vi "ADIS16448 Loop.vi"(8 "error in":errorcluster) -> ()   [LabVIEW 2019]
uses:
  Typedef/ADIS16448 Device Reference.ctl
  Typedef/ADIS16448 Hardware Configuration.ctl
  <vilib>/Rock Robotics/WPI/SPI/WPI_SPIMode.ctl
  <vilib>/Rock Robotics/SystemInterfaces/DIO/FPGA_DIOChannel.ctl
  <vilib>/Rock Robotics/SystemInterfaces/spilib/spi_bus.ctl
  Typedef/ADIS16448 Status.ctl
  Typedef/ADIS16448 Data.ctl
  Typedef/ADIS16448 Process.ctl
  Typedef/ADIS16448 Command Type.ctl
  <vilib>/Rock Robotics/SystemInterfaces/CounterEncoderSourceConvertion/FPGA_CounterEncoderSourceConvertionLVSourceType.ctl
  <vilib>/Rock Robotics/SystemInterfaces/DIO/FPGA_DIODigitalSourceChannel.ctl
  <vilib>/Rock Robotics/SystemInterfaces/AnalogTrigger/FPGA_AnalogTriggerIndex.ctl
  <vilib>/Rock Robotics/SystemInterfaces/AnalogTrigger/FPGA_AnalogTriggerOutType.ctl
  Typedef/ADIS16448 Calibration Time.ctl
  <vilib>/Rock Robotics/WPI/SPI/WPI_SPIDevRef.ctl
  Typedef/ADIS16448 Register.ctl
  <vilib>/Rock Robotics/WPI/Counter/WPI_CounterDigitalInputToDigitalSource.vi
  <vilib>/Rock Robotics/SystemInterfaces/Utilities/FPGA_UtilitiesRead LocalTime.vi
  <vilib>/ptbypt/NI_PtbyPt.lvlib
panel:
  in  "Calibration Time":T1
  in  "element":T2
  out "Waveform Chart":dbl(graph)
  in  "ADIS16448DevRef":T3={"DevStatus"={"status"=FALSE, "code"=0, "source"=""}, "Hardware Config"={"SPI Clock Rate (Hz)"=1000000.0, "IMU SPI Mode (3)"=enum."Mode 3 (Clk Idle High,Sample on Trailing)", "IMU Reset Pin"=enum."SPI Port CS2", "IMU SPI Bus"=enum."SPI On-Board, CS0", "IMU Data Ready Pin"=enum."SPI Port CS1", "Stall Config"={"Pow2BytesPerRead"=255, "StallTicks"=640, "CsToSclkTicks"=5}, "IMU Status LED Pin"=enum."DIO MXP 9"}, "Calibration Complete"=refnum, "Status FIFO"=refnum, "Last Value Reference"=refnum, "Sychronous Process VI"=refnum, "Cmd FIFO"=refnum, "Source"={"DevStatus"={"status"=FALSE, "code"=0, "source"=""}, "AnalogTriggerMode?"=FALSE, "DigitalMode"={"DIO Channel"=enum."Disabled"}, "AnalogTriggerMode"={"AnalogTriggerIndex"=enum."Trig 0", "OutputType"=enum."InWindow"}}, "Data FIFO"=refnum, "IMU Status LED Pin"=enum."DIO MXP 9", "Calibration Time"=5}
  in  "Main Name":string
  # "XG_BIAS_LOW"
  # "XG_BIAS_HIGH"
  # "YG_BIAS_LOW"
  # "YG_BIAS_HIGH"
  # "ZG_BIAS_LOW"
  # "ZG_BIAS_HIGH"
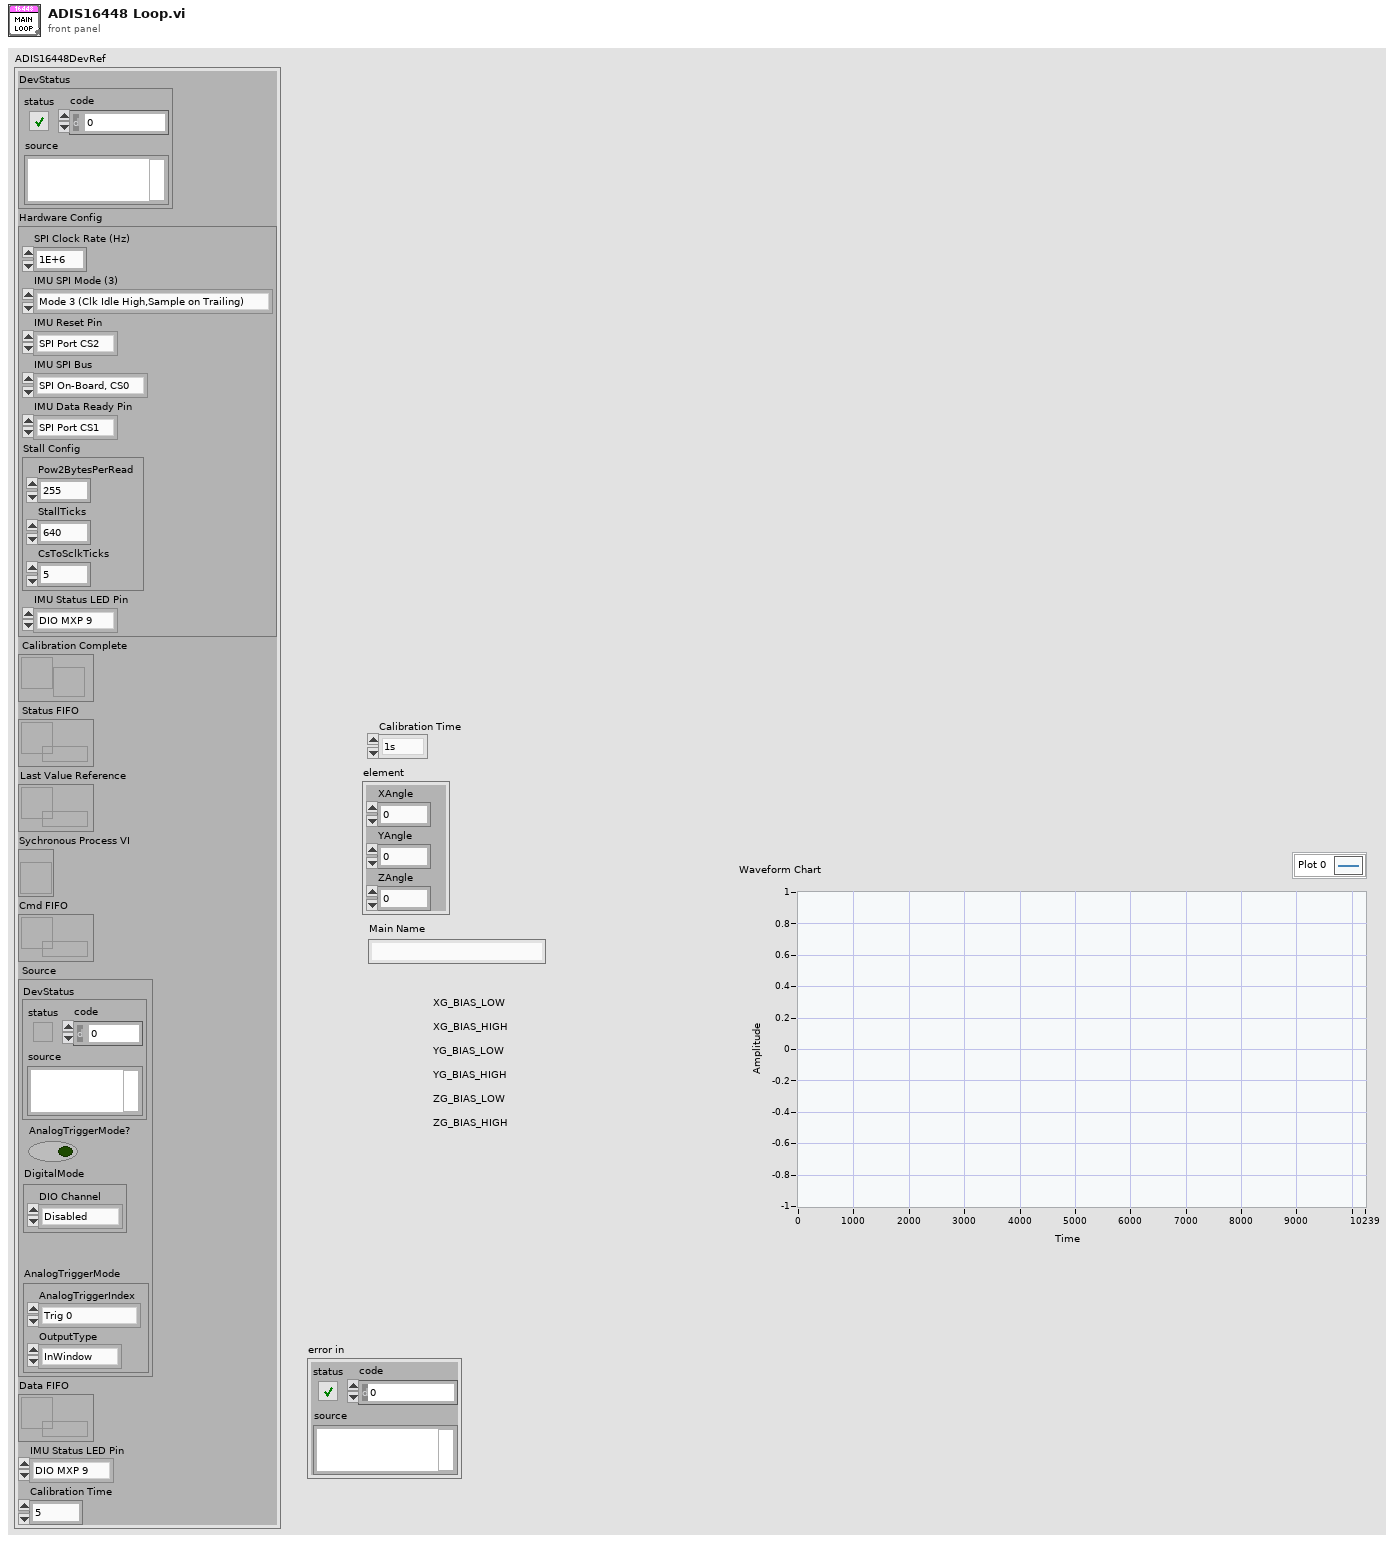
[diagram p1: front panel]
types:
  T1 = typedef "ADIS16448 Calibration Time.ctl" = enum16{"1s", "s", "4.9ms", "9.8ms", "19.5ms", "39.1ms", "78.1ms", "156.3ms", "312.5ms", "625ms", "1.25s", "2.5s", "5s", "10s", "20s", "40s", "80s", "160s", "320s"}
  T2 = typedef "ADIS16448 Data.ctl" = cluster{"XAngle":dbl, "YAngle":dbl, "ZAngle":dbl}
  T3 = typedef "ADIS16448 Device Reference.ctl" = cluster{"DevStatus":errorcluster, "Hardware Config":T4, "Calibration Complete":refnum<notifier>, "Status FIFO":refnum<k33>, "Last Value Reference":refnum<data-value>, "Sychronous Process VI":T8, "Cmd FIFO":refnum<k33>, "Source":T9, "Data FIFO":refnum<k33>, "IMU Status LED Pin":T6, "Calibration Time":i32}
  T4 = typedef "ADIS16448 Hardware Configuration.ctl" = cluster{"SPI Clock Rate (Hz)":dbl, "IMU SPI Mode (3)":T5, "IMU Reset Pin":T6, "IMU SPI Bus":T7, "IMU Data Ready Pin":T6, "Stall Config":cluster{"Pow2BytesPerRead":u8, "StallTicks":u16, "CsToSclkTicks":u8}, "IMU Status LED Pin":T6}
  T5 = typedef "WPI_SPIMode.ctl" = enum16{"Mode 0 (Clk Idle Low,Sample on Leading)", "Mode 1 (Clk Idle Low,Sample on Trailing)", "Mode 2 (Clk Idle High,Sample on Leading)", "Mode 3 (Clk Idle High,Sample on Trailing)"}
  T6 = typedef "FPGA_DIOChannel.ctl" = enum8{"DIO 0", "DIO 1", "DIO 2", "DIO 3", "DIO 4", "DIO 5", "DIO 6", "DIO 7", "DIO 8", "DIO 9", "DIO MXP 0", "DIO MXP 1", "DIO MXP 2", "DIO MXP 3", "DIO MXP 4", "DIO MXP 5", "DIO MXP 6", "DIO MXP 7", "DIO MXP 8", "DIO MXP 9", "DIO MXP 10", "DIO MXP 11", "DIO MXP 12", "DIO MXP 13", "DIO MXP 14", "DIO MXP 15", "SPI Port CS1", "SPI Port CS2", "SPI Port CS3", "SPI Port MISO", "SPI Port MOSI", "Invalid"}
  T7 = typedef "spi_bus.ctl" = enum16{"SPI On-Board, CS0", "SPI On-Board, CS1", "SPI On-Board, CS2", "SPI On-Board, CS3", "SPI MXP", "Invalid"}
  T8 = typedef "ADIS16448 Process.ctl" = refnum<vi>
  T9 = typedef "FPGA_CounterEncoderSourceConvertionLVSourceType.ctl" = cluster{"DevStatus":errorcluster, "AnalogTriggerMode?":bool, "DigitalMode":cluster{"DIO Channel":T10}, "AnalogTriggerMode":cluster{"AnalogTriggerIndex":T11, "OutputType":T12}}
  T10 = typedef "FPGA_DIODigitalSourceChannel.ctl" = enum8{"DIO 0", "DIO 1", "DIO 2", "DIO 3", "DIO 4", "DIO 5", "DIO 6", "DIO 7", "DIO 8", "DIO 9", "DIO MXP 0", "DIO MXP 1", "DIO MXP 2", "DIO MXP 3", "DIO MXP 4", "DIO MXP 5", "DIO MXP 6", "DIO MXP 7", "DIO MXP 8", "DIO MXP 9", "DIO MXP 10", "DIO MXP 11", "DIO MXP 12", "DIO MXP 13", "DIO MXP 14", "DIO MXP 15", "SPI Port CS1", "SPI Port CS2", "SPI Port CS3", "SPI Port MISO", "SPI Port MOSI", "Disabled"}
  T11 = typedef "FPGA_AnalogTriggerIndex.ctl" = enum8{"Trig 0", "Trig 1", "Trig 2", "Trig 3", "Trig 4", "Trig 5", "Trig 6", "Trig 7", "Invalid"}
  T12 = typedef "FPGA_AnalogTriggerOutType.ctl" = enum16{"InWindow", "TriggerState", "Rising", "Falling"}
  T13 = typedef "WPI_SPIDevRef.ctl" = cluster{"DevStatus":errorcluster, "Handle":i32, "SPI Bus":T7}
  T14 = cluster{"SPIDevRef":T13, "Data Counter":u16, "Reset":bool, "Digital Source":T9, "Bytes Per Sample":u32, "Data":dbl[], "ADIS16448DevRef":T3, "TimeStampPrev":u32, "Sensor to Robot Rotation":dbl[][], "AutoSPI Active?":bool, "Offsets":dbl[], "Offset Counter":i32, "Data Header":u8[], "Zero Byte Count":u8, "AutoSPI Override":bool}
  T15 = typedef "ADIS16448 Status.ctl" = cluster{"Calibrated?":bool}
  T16 = typedef "ADIS16448 Register.ctl" = u8
  T17 = typedef "ADIS16448 Command Type.ctl" = cluster{"Command":enum16{"None", "Reset", "Rewrite Config", "Start Recal", "Recalibrate", "Recal Complete", "Exit Auto SPI", "Start Auto SPI"}, "Data":u32}
  T18 = typedef "WPI_DigitalOutputDevRef.ctl" = cluster{"DIO Channel":T6, "DevStatus":errorcluster}
  T19 = typedef "WPI_DigitalInputDevRef.ctl" = cluster{"DevStatus":errorcluster, "DIO Channel":T6}
  T20 = cluster{"Pow2BytesPerRead":u8, "StallTicks":u16, "CsToSclkTicks":u8}
  T21 = enum16{"None", "Reset", "Rewrite Config", "Start Recal", "Recalibrate", "Recal Complete", "Exit Auto SPI", "Start Auto SPI"}
  T22 = enum32{"Bad", "Idle", "Run top level", "Running"}
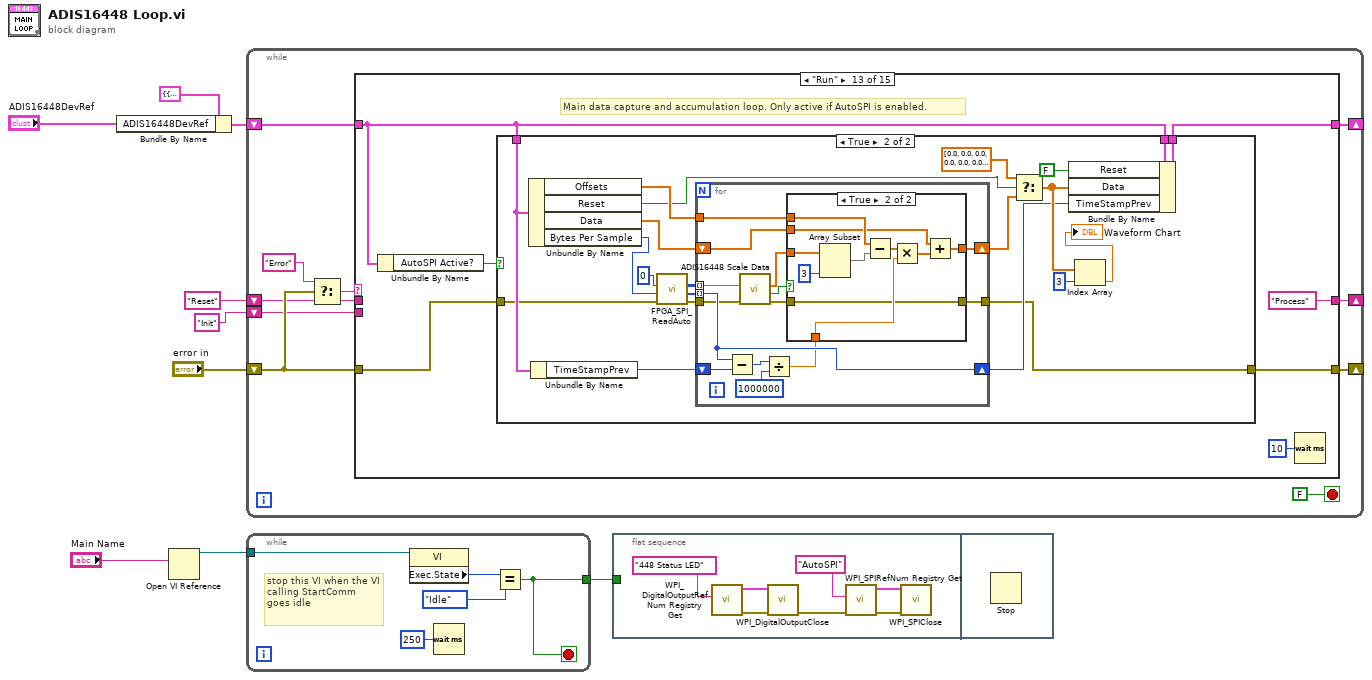
[diagram p0: block diagram]
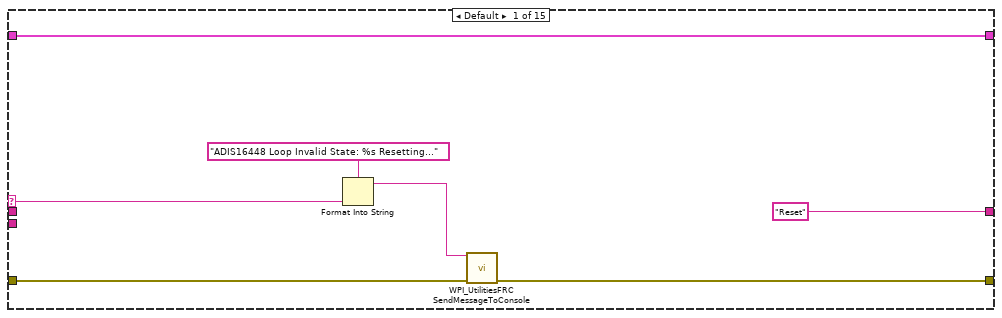
[diagram p2: hidden frame]
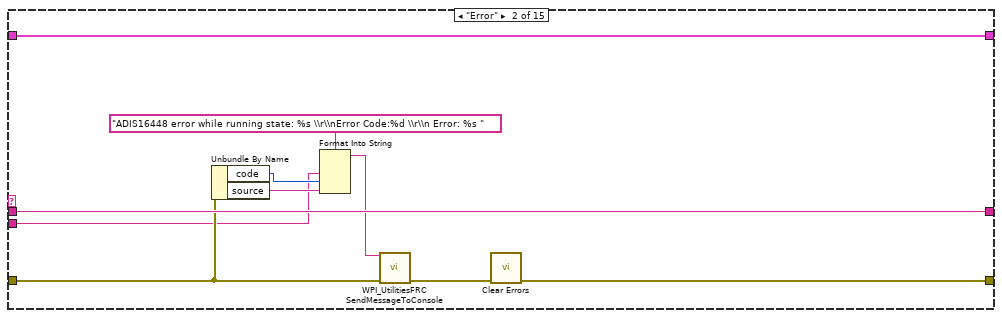
[diagram p3: hidden frame]
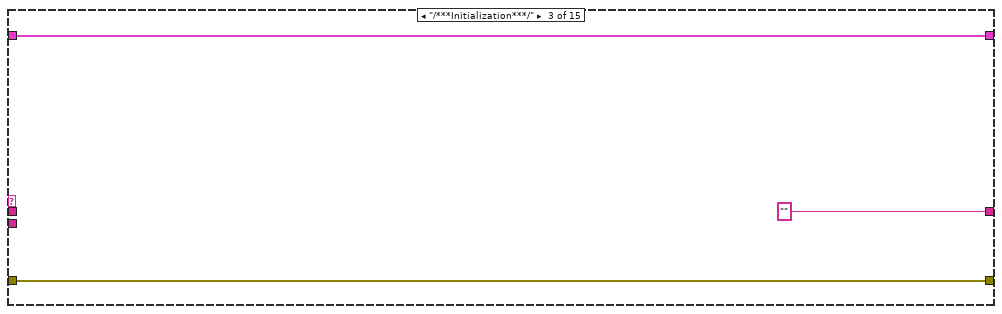
[diagram p4: hidden frame]
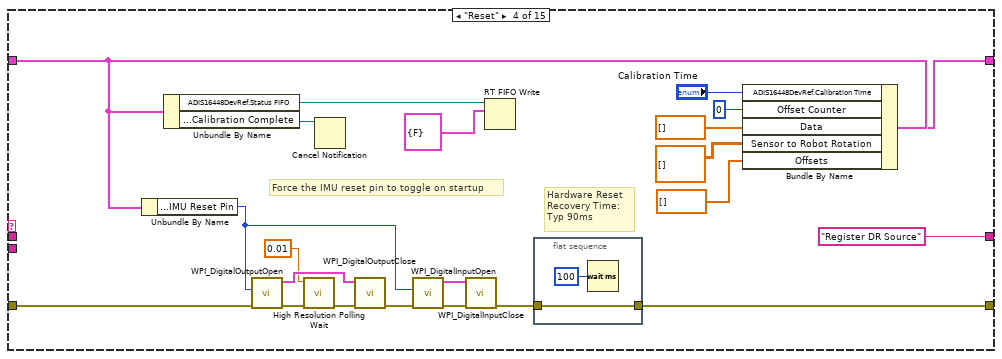
[diagram p5: hidden frame]
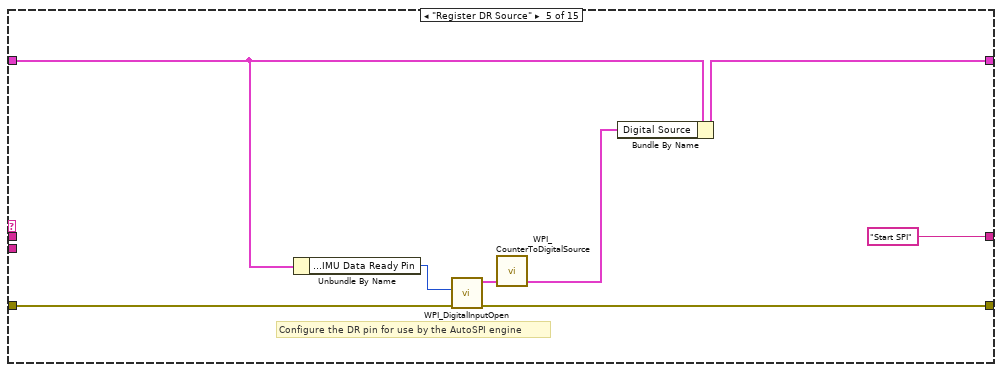
[diagram p6: hidden frame]
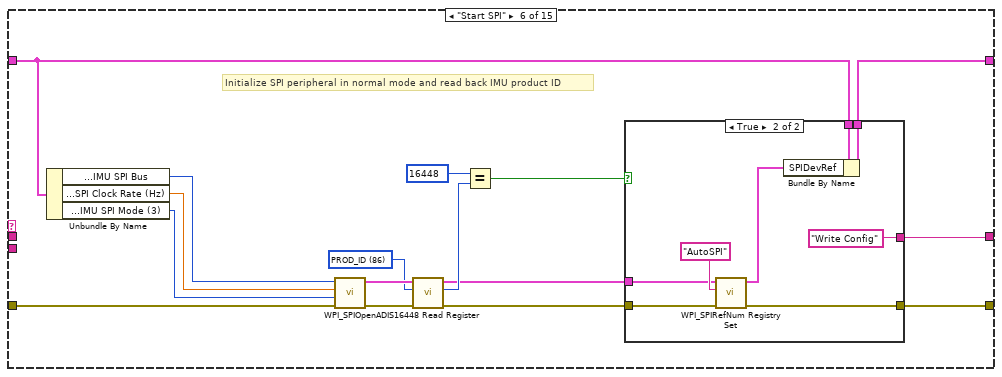
[diagram p7: hidden frame]
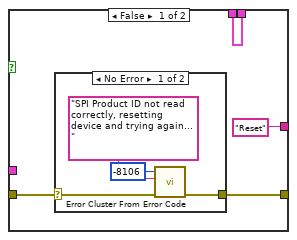
[diagram p8: hidden frame]
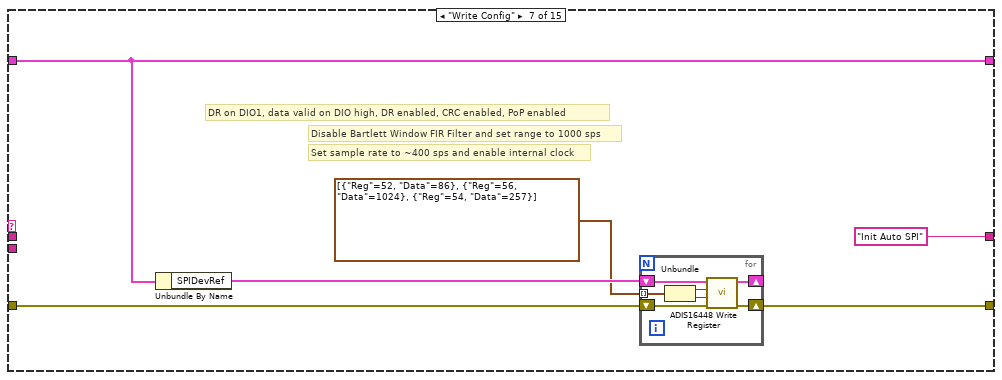
[diagram p10: hidden frame]
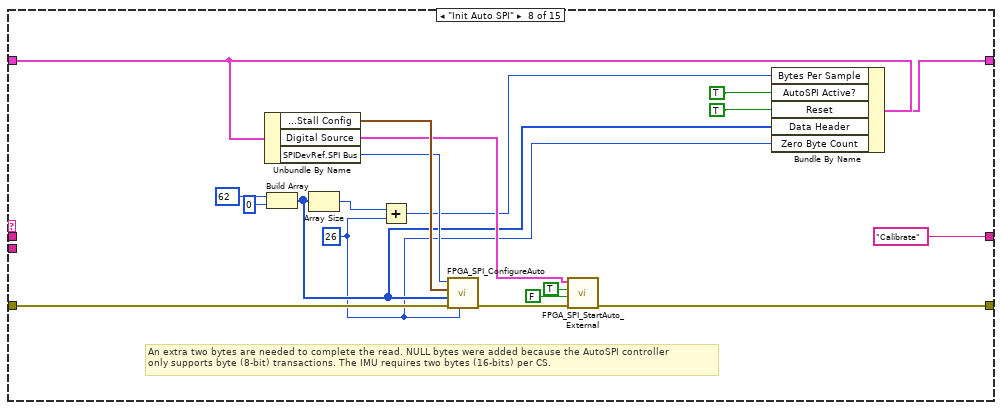
[diagram p11: hidden frame]
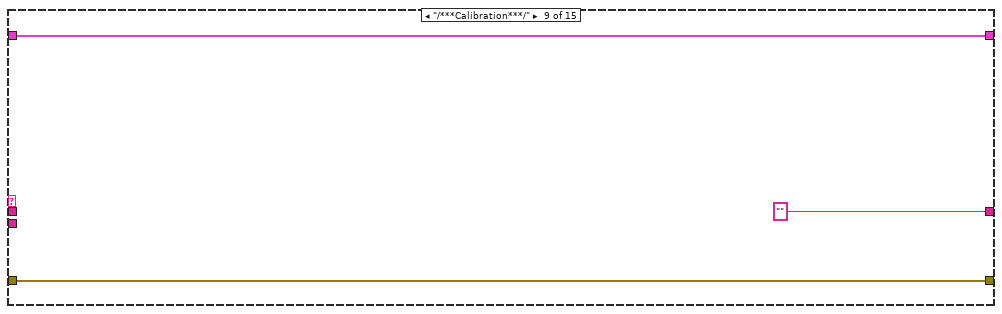
[diagram p12: hidden frame]
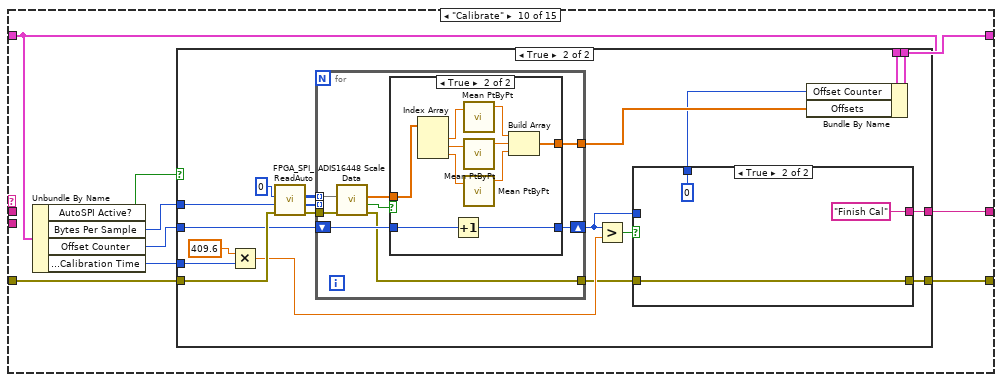
[diagram p13: hidden frame]
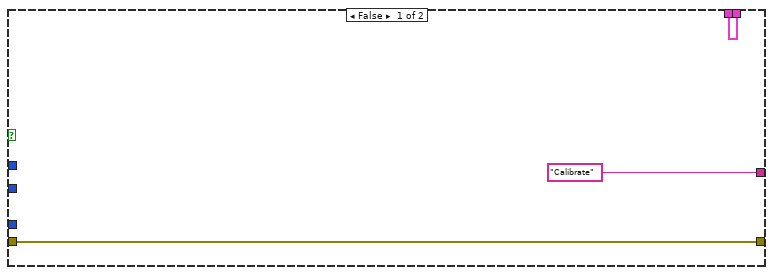
[diagram p14: hidden frame]
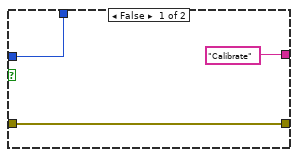
[diagram p15: hidden frame]
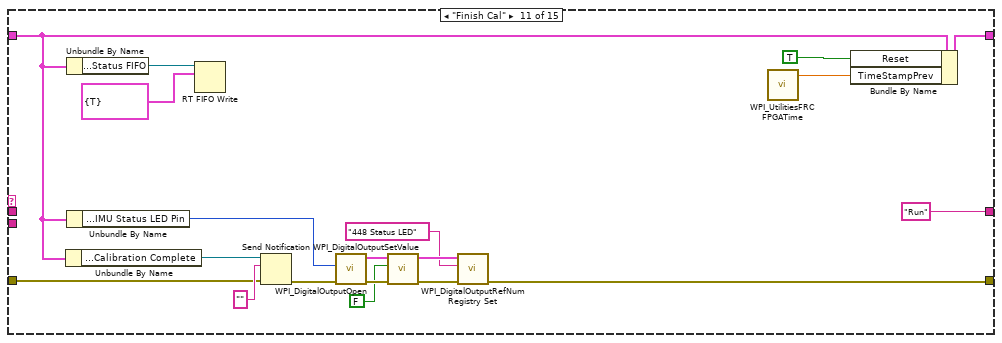
[diagram p17: hidden frame]
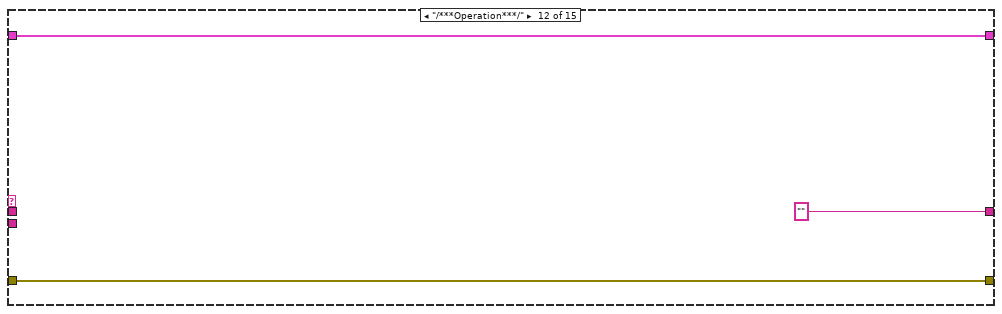
[diagram p18: hidden frame]
diagram:
  n1 = Bundle By Name(cluster=T14 {"SPIDevRef"={"DevStatus"={"status"=FALSE, "code"=0, "source"=""}, "Handle"=0, "SPI Bus"=enum."SPI On-Board, CS0"}, "Data Counter"=0, "Reset"=FALSE, "Digital Source"={"DevStatus"={"status"=FALSE, "code"=0, "source"=""}, "AnalogTriggerMode?"=FALSE, "DigitalMode"={"DIO Channel"=enum."DIO 1"}, "AnalogTriggerMode"={"AnalogTriggerIndex"=enum."Trig 0", "OutputType"=enum."InWindow"}}, "Bytes Per Sample"=0, "Data"=[0.0, 0.0, 0.0, 0.0, 0.0, 0.0, 0.0, 0.0], "ADIS16448DevRef"={"DevStatus"={"status"=FALSE, "code"=0, "source"=""}, "Hardware Config"={"SPI Clock Rate (Hz)"=1000000.0, "IMU SPI Mode (3)"=enum."Mode 3 (Clk Idle High,Sample on Trailing)", "IMU Reset Pin"=enum."SPI Port CS2", "IMU SPI Bus"=enum."SPI On-Board, CS0", "IMU Data Ready Pin"=enum."SPI Port CS1", "Stall Config"={"Pow2BytesPerRead"=255, "StallTicks"=640, "CsToSclkTicks"=5}, "IMU Status LED Pin"=enum."DIO MXP 9"}, "Calibration Complete"=refnum, "Status FIFO"=refnum, "Last Value Reference"=refnum, "Sychronous Process VI"=refnum, "Cmd FIFO"=refnum, "Source"={"DevStatus"={"status"=FALSE, "code"=0, "source"=""}, "AnalogTriggerMode?"=FALSE, "DigitalMode"={"DIO Channel"=enum."Disabled"}, "AnalogTriggerMode"={"AnalogTriggerIndex"=enum."Trig 0", "OutputType"=enum."InWindow"}}, "Data FIFO"=refnum, "IMU Status LED Pin"=enum."DIO MXP 9", "Calibration Time"=5}, "TimeStampPrev"=0, "Sensor to Robot Rotation"=[], "AutoSPI Active?"=TRUE, "Offsets"=[0.0, 0.0, 0.0, 0.0, 0.0, 0.0, 0.0, 0.0], "Offset Counter"=0, "Data Header"=[], "Zero Byte Count"=0, "AutoSPI Override"=TRUE}, "ADIS16448DevRef"="ADIS16448DevRef") -> (w5:T14)
  n2 = Open VI Reference(vi path="Main Name") -> (vi reference=w8:refnum<vi>)  [unwired: 3 in, 3 out]
  n3 = while {
    shift-right: [w15] -> _
    shift-left: "Reset" -> [w12]
    shift-right: [w17] -> _
    shift-left: w5 -> [w18]
    shift-right: [w16] -> _
    shift-left: "error in" -> [w14]
    shift-left: "Init" -> [w10]
    stop <- FALSE stop-if-true
    n4 = Select(t="Error", s=w14, f=w12) -> (s? t:f=w13:string)
    n5 = case shown="\"Run\"" w13 {
      selector: w13 -> [w25 _ _ _ _ _ _ _ _ _ _ _ _ _ _]
      tunnel: w18 -> [w26 w36 w39 w56 w67 w80 w106 w131 w139 w140 w206 w218 w220 w286 w295]
      tunnel: [w26 w36 w39 w55 w70 w81 w106 w130 w139 w145 w214 w218 w224 w286 w302] -> w17
      tunnel: w14 -> [w24 w32 w38 w48 w69 w87 w108 w135 w138 w147 w207 w217 w223 w284 w304]
      tunnel: [w23 w33 w38 w60 w64 w79 w107 w118 w138 w146 w199 w217 w222 w283 w303] -> w16
      tunnel: ["Reset" w35 "" "Register DR Source" "Start SPI" w82 "Init Auto SPI" "Calibrate" "" w141 "Run" "" "Process" "Run Cmds" "Run"] -> w15
      tunnel: w12 -> [_ w35 _ _ _ _ _ _ _ _ _ _ _ _ _]
      tunnel: w10 -> [_ w27 _ _ _ _ _ _ _ _ _ _ _ _ _]
      frame Default {
        n6 = Format Into String(format string="ADIS16448 Loop Invalid State: %s Resetting...", w25) -> (resulting string=w22:string)  [unwired: 2 in, 1 out]
        n7 = call <vilib>:"WPI_UtilitiesFRC SendMessageToConsole.vi"("Message"=w22, "error in (no error)"=w24) -> ("error out"=w23:errorcluster)  [unwired: 13 in]
      }
      frame "Error" {
        n8 = Unbundle By Name(w32) -> ("code"=w29:i32, "source"=w28:string)
        n9 = Format Into String(format string="ADIS16448 error while running state: %s \\r\\nError Code:%d \\r\\n Error: %s ", w27, w29, w28) -> (resulting string=w31:string)  [unwired: 2 in, 1 out]
        n10 = call <vilib>:"WPI_UtilitiesFRC SendMessageToConsole.vi"("Message"=w31, "error in (no error)"=w32) -> ("error out"=w34:errorcluster)  [unwired: 13 in]
        n11 = call <vilib>:"Clear Errors.vi"("error in (no error)"=w34) -> ("error out"=w33:errorcluster)  [unwired: 5 in, 1 out]
      }
      frame "/***Initialization***/" {
      }
      frame "Reset" {
        # "Hardware Reset Recovery Time: Typ 90ms"
        # "Force the IMU reset pin to toggle on startup"
        n12 = Unbundle By Name(w56) -> ("ADIS16448DevRef.Hardware Config.IMU Reset Pin"=w44:T6)
        n13 = Unbundle By Name(w56) -> ("ADIS16448DevRef.Status FIFO"=w58:refnum<k33>, "ADIS16448DevRef.Calibration Complete"=w59:refnum<notifier>)
        n14 = call <vilib>:"WPI_DigitalOutputOpen.vi"("error in (no error)"=w48, "DIO Channel"=w44) -> ("error out"=w46:errorcluster, "DigitalOutputDevRef"=w53:T18)  [unwired: 8 in]
        n15 = call <vilib>:"High Resolution Polling Wait.vi"("error in (no error)"=w46, "seconds to wait"=0.01) -> ("error out"=w47:errorcluster)  [unwired: 9 in]
        n16 = Cancel Notification(0:w59) -> ()  [unwired: 1 in, 3 out]
        n17 = call <vilib>:"WPI_DigitalOutputClose.vi"("error in (no error)"=w47, "DigitalOutputDevRef"=w53) -> ("error out"=w50:errorcluster)  [unwired: 9 in]
        n18 = call <vilib>:"WPI_DigitalInputOpen.vi"("error in (no error)"=w50, "DIO Channel"=w44) -> ("error out"=w51:errorcluster, "DigitalInputDevRef"=w52:T19)  [unwired: 8 in]
        n19 = call <vilib>:"WPI_DigitalInputClose.vi"("error in (no error)"=w51, "DigitalInputDevRef"=w52) -> ("error out"=w49:errorcluster)  [unwired: 9 in]
        n20 = RT FIFO Write(0:w58, 1:T15 {"Calibrated?"=FALSE} ("element")) -> ()  [unwired: 3 in, 4 out]
        n21 = flat-sequence {
          tunnel: [w63] -> w60
          tunnel: w49 -> [w63]
          frame #0 {
            n22 = Wait (ms)(milliseconds to wait=u32 100) -> ()  [unwired: 1 out]
          }
        }
        n23 = Bundle By Name(cluster=w56, "ADIS16448DevRef.Calibration Time"="Calibration Time", "Offset Counter"=u32 0, "Data"=dbl[] [], "Sensor to Robot Rotation"=dbl[][] [], "Offsets"=dbl[] []) -> (w55:T14)
      }
      frame "Register DR Source" {
        # "Configure the DR pin for use by the AutoSPI engine"
        n24 = Unbundle By Name(w67) -> ("ADIS16448DevRef.Hardware Config.IMU Data Ready Pin"=w66:T6)
        n25 = call <vilib>:"WPI_DigitalInputOpen.vi"("error in (no error)"=w69, "DIO Channel"=w66) -> ("error out"=w64:errorcluster, "DigitalInputDevRef"=w68:T19)  [unwired: 8 in]
        n26 = call-poly <vilib>:"WPI_CounterToDigitalSource.vi"("DigitalInputDevRef"=w68) -> ("Digital Source"=w65:T9)  [unwired: 6 in]
        n27 = Bundle By Name(cluster=w67, "Digital Source"=w65) -> (w70:T14)
      }
      frame "Start SPI" {
        w72 = T16 86 items=["FLASH_CNT"=0, "Reserved 1"=2, "XGYRO_OUT"=4, "YGYRO_OUT"=6, "ZGYRO_OUT"=8, "XACCL_OUT"=10, "YACCL_OUT"=12, "ZACCL_OUT"=14, "XMAGN_OUT"=16, "YMAGN_OUT"=18, "ZMAGN_OUT"=20, "BARO_OUT"=22, "TEMP_OUT"=24, "XGYRO_OFF"=26, "YGYRO_OFF"=28, "ZGYRO_OFF"=30, "XACCL_OFF"=32, "YACCL_OFF"=34, "ZACCL_OFF"=36, "XMAGN_HIC"=38, "YMAGN_HIC"=40, "ZMAGN_HIC"=42, "XMAGN_SIC"=44, "YMAGN_SIC"=46, "ZMAGN_SIC"=48, "GPIO_CTRL"=50, "MSC_CTRL"=52, "SMPL_PRD"=54, "SENS_AVG"=56, "SEQ_CNT"=58, "DIAG_STAT"=60, "GLOB_CMD"=62, "ALM_MAG1"=64, "ALM_MAG2"=66, "ALM_SMPL1"=68, "ALM_SMPL2"=70, "ALM_CTRL"=72, "Reserved 2"=74, "Reserved 3"=76, "Reserved 4"=78, "Reserved 5"=80, "LOT_ID1"=82, "LOT_ID2"=84, "PROD_ID"=86, "SERIAL_NUM"=88] ("ADIS16448 Register")
        # "Initialize SPI peripheral in normal mode and read back IMU product ID"
        n28 = Unbundle By Name(w80) -> ("ADIS16448DevRef.Hardware Config.IMU SPI Bus"=w83:T7, "ADIS16448DevRef.Hardware Config.SPI Clock Rate (Hz)"=w84:dbl, "ADIS16448DevRef.Hardware Config.IMU SPI Mode (3)"=w85:T5)
        n29 = call <vilib>:"WPI_SPIOpen.vi"("error in"=w87, "Mode (3)"=w85, "Clock Rate (Hz)"=w84, "SPI Bus"=w83) -> ("error out"=w76:errorcluster, "SPIDevRef"=w75:T13)  [unwired: 6 in]
        n30 = call "ADIS16448 Read Register.vi"("error in (no error)"=w76, "ADIS16448 Register"=w72, "SPIDevRef in"=w75) -> ("error out"=w77:errorcluster, "Register Value"=w78:u16, "SPIDevRef out"=w74:T13)  [unwired: 6 in]
        n31 = Equal?(x=u16 16448 ("y"), y=w78) -> (x = y?=w86:bool)
        n32 = case shown="True" w86 {
          tunnel: ["Reset" "Write Config"] -> w82
          tunnel: w80 -> [w90 w103]
          tunnel: [w90 w102] -> w81
          tunnel: [w89 w97] -> w79
          tunnel: w77 -> [w88 w98]
          tunnel: w74 -> [_ w99]
          frame False {
            n33 = case shown="No Error" w88 {
              selector: w88 -> [w94 w96]
              tunnel: [w95 w96] -> w89
              frame No Error {
                n34 = call <vilib>:"Error Cluster From Error Code.vi"("error in (no error)"=w94, "error message (\"\")"="SPI Product ID not read correctly, resetting device and trying again..." ("error message (\"\")"), "error code (0)"=-8106) -> ("error out"=w95:errorcluster)  [unwired: 6 in]
              }
              frame Error {
              }
            }
          }
          frame True {
            n35 = call <vilib>:"WPI_SPIRefNum Registry Set.vi"("error in (no error)"=w98, "refnum name"="AutoSPI", "SPIDevRef"=w99) -> ("error out"=w97:errorcluster, "SPIDevRef"=w101:T13)  [unwired: 7 in]
            n36 = Bundle By Name(cluster=w103, "SPIDevRef"=w101) -> (w102:T14)
          }
        }
      }
      frame "Write Config" {
        # "DR on DIO1, data valid on DIO high, DR enabled, CRC enabled, PoP enabled"
        # "Set sample rate to ~400 sps and enable internal clock"
        # "Disable Bartlett Window FIR Filter and set range to 1000 sps"
        n37 = Unbundle By Name(w106) -> ("SPIDevRef"=w109:T13)
        n38 = for {
          tunnel: cluster{"Reg":T16, "Data":u16}[] [{"Reg"=52, "Data"=86}, {"Reg"=56, "Data"=1024}, {"Reg"=54, "Data"=257}] -> [w117] mode=indexing
          shift-right: [w113] -> w107
          shift-left: w108 -> [w112]
          shift-right: [w111] -> _
          shift-left: w109 -> [w114]
          n39 = Unbundle(w117) -> ("Reg"=w116:T16, "Data"=w115:u16)
          n40 = call "ADIS16448 Write Register.vi"("error in (no error)"=w112, "Data"=w115, "Register"=w116, "SPIDevRef in"=w114) -> ("error out"=w113:errorcluster, "SPIDevRef out"=w111:T13)  [unwired: 6 in]
        }
      }
      frame "Init Auto SPI" {
        w119 = u8 26 ("dimension size")
        # "An extra two bytes are needed to complete the read. NULL bytes were added because the AutoSPI controller \nonly supports byte (8-bit) transactions. The IMU requires two bytes (16-bits) per CS."
        n41 = Unbundle By Name(w131) -> ("ADIS16448DevRef.Hardware Config.Stall Config"=w129:T20, "Digital Source"=w127:T9, "SPIDevRef.SPI Bus"=w126:T7)
        n42 = Build Array(u8 62 ("hi"), u8 0 ("element")) -> (w120:u8[])
        n43 = Array Size(array=w120) -> (size(s)=w124:i32)
        n44 = Add(x=w124, y=w119) -> (x+y=w121:i32)
        n45 = call <vilib>:"FPGA_SPI_ConfigureAuto.vi"("SPI Auto Zero Byte Count"=w119, "error in"=w135, "SPI Auto TX Byte Array"=w120, "Stall Config"=w129, "SPI Bus"=w126) -> ("error out"=w134:errorcluster)  [unwired: 6 in]
        n46 = call <vilib>:"FPGA_SPI_StartAuto_External.vi"("error in (no error)"=w134, "Falling Edge"=FALSE, "Rising Edge"=TRUE, "Source"=w127) -> ("error out"=w118:errorcluster)  [unwired: 7 in]
        n47 = Bundle By Name(cluster=w131, "Bytes Per Sample"=w121, "AutoSPI Active?"=TRUE, "Reset"=TRUE, "Data Header"=w120, "Zero Byte Count"=w119) -> (w130:T14)
      }
      frame "/***Calibration***/" {
      }
      frame "Calibrate" {
        n48 = Unbundle By Name(w140) -> ("AutoSPI Active?"=w148:bool, "Bytes Per Sample"=w144:u32, "Offset Counter"=w143:i32, "ADIS16448DevRef.Calibration Time"=w142:i32)
        n49 = case shown="True" w148 {
          tunnel: [w151 w170] -> w145
          tunnel: w147 -> [w150 w165]
          tunnel: [w150 w153] -> w146
          tunnel: w140 -> [w151 w166]
          tunnel: w144 -> [_ w163]
          tunnel: w143 -> [_ w160]
          tunnel: w142 -> [_ w161]
          tunnel: ["Calibrate" w155] -> w141
          frame False {
          }
          frame True {
            n50 = Multiply(x=409.6, y=w161) -> (x*y=w154:dbl)
            n51 = call <vilib>:"FPGA_SPI_ReadAuto.vi"("error in (no error)"=w165, "Bytes per Sample"=w163, "Samples to Read"=u32 0) -> ("error out"=w164:errorcluster, "Timestamps"=w167:u32[], "Data"=w168:u8[][])  [unwired: 6 in]
            n52 = for {
              tunnel: w168 -> [w184] mode=indexing
              tunnel: w167 -> [_] mode=indexing
              tunnel: w164 -> [w183]
              tunnel: [w178] -> w158
              tunnel: [w177] -> w152
              shift-right: [w179] -> w157
              shift-left: w160 -> [w180]
              n53 = call "ADIS16448 Scale Data.vi"("error in (no error)"=w183, "New Data In"=w184) -> ("error out"=w177:errorcluster, "Data Good?"=w182:bool, "Data Out"=w181:dbl[])  [unwired: 7 in]
              n54 = case shown="True" w182 {
                tunnel: w181 -> [w186 w188]
                tunnel: [w186 w187] -> w178
                tunnel: w180 -> [w185 w196]
                tunnel: [w185 w195] -> w179
                frame False {
                }
                frame True {
                  n55 = Index Array(array=w188) -> (element #1=w189:dbl, element #2=w190:dbl, element #3=w191:dbl)  [unwired: 3 in]
                  n56 = Increment(x=w196) -> (x+1=w195:i32)
                  n57 = call <vilib>:"Mean PtByPt.vi"("x"=w189) -> ("mean"=w192:dbl)  [unwired: 3 in, 1 out]
                  n58 = call <vilib>:"Mean PtByPt.vi"("x"=w190) -> ("mean"=w193:dbl)  [unwired: 3 in, 1 out]
                  n59 = call <vilib>:"Mean PtByPt.vi"("x"=w191) -> ("mean"=w194:dbl)  [unwired: 3 in, 1 out]
                  n60 = Build Array(w192, w193, w194) -> (w187:dbl[])
                }
              }
            }
            n61 = Greater?(x=w157, y=w154) -> (0:w159:bool)
            n62 = case shown="True" w159 {
              tunnel: w157 -> [w173 _]
              tunnel: [w173 u32 0 ("Offset Counter")] -> w156
              tunnel: ["Calibrate" "Finish Cal"] -> w155
              tunnel: [w171 w174] -> w153
              tunnel: w152 -> [w171 w174]
              frame False {
              }
              frame True {
              }
            }
            n63 = Bundle By Name(cluster=w166, "Offset Counter"=w156, "Offsets"=w158) -> (w170:T14)
          }
        }
      }
      frame "Finish Cal" {
        n64 = Unbundle By Name(w206) -> ("ADIS16448DevRef.Calibration Complete"=w212:refnum<notifier>)
        n65 = Unbundle By Name(w206) -> ("ADIS16448DevRef.Status FIFO"=w210:refnum<k33>)
        n66 = Unbundle By Name(w206) -> ("ADIS16448DevRef.Hardware Config.IMU Status LED Pin"=w197:T6)
        n67 = RT FIFO Write(0:w210, 1:T15 {"Calibrated?"=TRUE} ("element")) -> ()  [unwired: 3 in, 4 out]
        n68 = Send Notification(notification="", notifier=w212, error in (no error)=w207) -> (error out=w200:errorcluster)  [unwired: 1 out]
        n69 = call <vilib>:"WPI_DigitalOutputOpen.vi"("error in (no error)"=w200, "DIO Channel"=w197) -> ("error out"=w205:errorcluster, "DigitalOutputDevRef"=w204:T18)  [unwired: 8 in]
        n70 = call <vilib>:"WPI_DigitalOutputSetValue.vi"("error in (no error)"=w205, "Value"=FALSE, "DigitalOutputDevRef"=w204) -> ("error out"=w203:errorcluster, "DigitalOutputDevRef"=w202:T18)  [unwired: 7 in]
        n71 = call <vilib>:"WPI_DigitalOutputRefNum Registry Set.vi"("error in (no error)"=w203, "refnum name"="448 Status LED", "DigitalOutputDevRef"=w202) -> ("error out"=w199:errorcluster)  [unwired: 7 in, 1 out]
        n72 = call <vilib>:"WPI_UtilitiesFRC FPGATime.vi"() -> ("FPGA Time"=w208:dbl)  [unwired: 10 in, 1 out]
        n73 = Bundle By Name(cluster=w206, "Reset"=TRUE ("First Run"), "TimeStampPrev"=w208) -> (w214:T14)
      }
      frame "/***Operation***/" {
      }
      frame "Run" {
        # "Main data capture and accumulation loop. Only active if AutoSPI is enabled."
        n74 = Unbundle By Name(w220) -> ("AutoSPI Active?"=w219:bool)
        n75 = case shown="True" w219 {
          tunnel: [w227 w248] -> w224
          tunnel: w223 -> [w226 w232]
          tunnel: [w226 w228] -> w222
          tunnel: w220 -> [w227 w236]
          tunnel: w220 -> [_ w233]
          frame False {
          }
          frame True {
            n76 = Unbundle By Name(w233) -> ("Offsets"=w230:dbl[], "Reset"=w229:bool, "Data"=w242:dbl[], "Bytes Per Sample"=w246:u32)
            n77 = Unbundle By Name(w233) -> ("TimeStampPrev"=w235:u32)
            n78 = call <vilib>:"FPGA_SPI_ReadAuto.vi"("error in (no error)"=w232, "Bytes per Sample"=w246, "Samples to Read"=u32 0) -> ("error out"=w231:errorcluster, "Timestamps"=w243:u32[], "Data"=w244:u8[][])  [unwired: 6 in]
            n79 = for {
              tunnel: w244 -> [w260] mode=indexing
              tunnel: w243 -> [w261] mode=indexing
              shift-right: [w252] -> w241
              shift-left: w242 -> [w251]
              shift-right: [w261] -> w234
              shift-left: w235 -> [w262]
              tunnel: w231 -> [w259]
              tunnel: w230 -> [w256]
              tunnel: [w249] -> w228
              n80 = Subtract(x=w261, y=w262) -> (x-y=w255:u32)
              n81 = call "ADIS16448 Scale Data.vi"("error in (no error)"=w259, "New Data In"=w260) -> ("error out"=w250:errorcluster, "Data Good?"=w258:bool, "Data Out"=w257:dbl[])  [unwired: 7 in]
              n82 = Divide(x=w255, y=u32 1000000) -> (x/y=w253:dbl)
              n83 = case shown="True" w258 {
                tunnel: w257 -> [_ w273]
                tunnel: w256 -> [_ w271]
                tunnel: w253 -> [_ w269]
                tunnel: [w264 w268] -> w252
                tunnel: w251 -> [w264 w266]
                tunnel: w250 -> [w263 w265]
                tunnel: [w263 w265] -> w249
                frame False {
                }
                frame True {
                  n84 = Array Subset(array=w273, length=3) -> (w272:dbl[])  [unwired: 1 in]
                  n85 = Subtract(x=w271, y=w272) -> (x-y=w270:dbl[])
                  n86 = Multiply(x=w270, y=w269) -> (x*y=w267:dbl[])
                  n87 = Add(x=w266, y=w267) -> (x+y=w268:dbl[])
                }
              }
            }
            n88 = Select(t=dbl[] [0.0, 0.0, 0.0, 0.0, 0.0, 0.0, 0.0, 0.0] ("Angle and Vel"), s=w229, f=w241) -> (s? t:f=w239:dbl[])
            n89 = Bundle By Name(cluster=w236, "Reset"=FALSE ("First Run"), "Data"=w239, "TimeStampPrev"=w234) -> (w248:T14)
            n90 = Index Array(array=w239, index=3) -> (element=→"Waveform Chart":dbl)
          }
        }
        n91 = Wait (ms)(milliseconds to wait=u32 10) -> ()  [unwired: 1 out]
      }
      frame "Process" {
        n92 = Unbundle By Name(w286) -> ("ADIS16448DevRef.Sychronous Process VI"=w281:T8, "ADIS16448DevRef.Data FIFO"=w285:refnum<k33>, "Data"=w280:dbl[])
        n93 = Index Array(array=w280) -> (element #1=w279:dbl, element #2=w278:dbl, element #3=w277:dbl)  [unwired: 3 in]
        n94 = Bundle By Name(cluster="element", "XAngle"=w279, "YAngle"=w278, "ZAngle"=w277) -> (w275:T2)
        n95 = RT FIFO Write(0:w285, 1:w275) -> ()  [unwired: 3 in, 4 out]
        n96 = Not A Number/Path/Refnum?(number/path/refnum=w281) -> (NaN/Path/Refnum?=w282:bool)
        n97 = case shown="False" w282 {
          tunnel: w284 -> [w288 w293]
          tunnel: w275 -> [_ _]
          tunnel: [w292 w293] -> w283
          tunnel: w281 -> [w291 _]
          frame False {
            n98 = call-by-ref "?"(reference=w291, error in=w288, 8:"error in (no error)"=w288) -> (error out=w289:errorcluster, 0:"error out"=w290:errorcluster)  [unwired: 10 in, 1 out]
            n99 = Merge Errors(w289, w290) -> (w292:errorcluster)
          }
          frame True {
          }
        }
      }
      frame "Run Cmds" {
        n100 = Unbundle By Name(w295) -> ("ADIS16448DevRef.Cmd FIFO"=w305:refnum<k33>)
        n101 = Unbundle By Name(w295) -> ("ADIS16448DevRef.Status FIFO"=w300:refnum<k33>, "ADIS16448DevRef.Calibration Complete"=w301:refnum<notifier>)
        n102 = RT FIFO Read(0:w305, 1:T17 {"Command"=enum."None", "Data"=0} ("element")) -> (8:w298:refnum<k33>, 9:w297:T17)  [unwired: 2 in, 3 out]
        n103 = Unbundle(w297) -> ("Command"=w294:T21, "Data"=w296:u32)
        n104 = case shown="\"Start Auto SPI\"" w294 {
          tunnel: w295 -> [w307 w312 w320 w329 w393 w407 w446 w461]
          tunnel: w304 -> [w308 w311 w318 w332 w398 w423 w456 w465]
          tunnel: [w308 w311 w317 w331 w398 w410 w447 w465] -> w303
          tunnel: [w307 w310 w320 w328 w392 w406 w446 w460] -> w302
          tunnel: w301 -> [_ _ _ _ w397 _ _ _]
          tunnel: w300 -> [_ _ _ _ w395 _ _ w463]
          tunnel: w298 -> [_ _ w315 w330 _ w421 w458 _]
          tunnel: w296 -> [_ _ _ _ _ _ _ _]
          tunnel: w295 -> [_ _ w314 w337 _ w404 w445 _]
          frame "None", Default {
          }
          frame "Reset" {
            n105 = Bundle By Name(cluster=w312, "Reset"=TRUE ("First Run")) -> (w310:T14)
          }
          frame "Rewrite Config" {
            n106 = Unbundle By Name(w314) -> ("SPIDevRef"=w313:T13)
            n107 = RT FIFO Write(0:w315, 1:T17 {"Command"=enum."Start Auto SPI", "Data"=0} ("element")) -> ()  [unwired: 3 in, 4 out]
            n108 = for {
              tunnel: cluster{"Reg":T16, "Data":u16}[] [{"Reg"=52, "Data"=86}, {"Reg"=56, "Data"=1024}, {"Reg"=54, "Data"=257}] -> [w327] mode=indexing
              shift-right: [w323] -> w317
              shift-left: w318 -> [w322]
              shift-right: [w321] -> _
              shift-left: w313 -> [w324]
              n109 = Unbundle(w327) -> ("Reg"=w326:T16, "Data"=w325:u16)
              n110 = call "ADIS16448 Write Register.vi"("error in (no error)"=w322, "Data"=w325, "Register"=w326, "SPIDevRef in"=w324) -> ("error out"=w323:errorcluster, "SPIDevRef out"=w321:T13)  [unwired: 6 in]
            }
          }
          frame "Recalibrate" {
            n111 = Unbundle By Name(w337) -> ("AutoSPI Override"=w336:bool, "Bytes Per Sample"=w335:u32, "Offset Counter"=w333:i32, "ADIS16448DevRef.Calibration Time"=w334:i32)
            n112 = case shown="True" w336 {
              tunnel: w335 -> [_ w356]
              tunnel: w334 -> [_ w354]
              tunnel: w333 -> [_ w353]
              tunnel: w332 -> [w341 w345]
              tunnel: [w341 w343] -> w331
              tunnel: w330 -> [w339 w346]
              tunnel: w329 -> [w338 w350]
              tunnel: [w338 w349] -> w328
              frame False {
                n113 = RT FIFO Write(0:w339, 1:T17 {"Command"=enum."Recalibrate", "Data"=0} ("element")) -> ()  [unwired: 3 in, 4 out]
              }
              frame True {
                n114 = call <vilib>:"FPGA_SPI_ReadAuto.vi"("error in (no error)"=w345, "Bytes per Sample"=w356, "Samples to Read"=u32 0) -> ("error out"=w358:errorcluster, "Timestamps"=w359:u32[], "Data"=w360:u8[][])  [unwired: 6 in]
                n115 = Multiply(x=409.6, y=w354) -> (x*y=w352:dbl)
                n116 = for {
                  tunnel: w360 -> [w376] mode=indexing
                  tunnel: w359 -> [_] mode=indexing
                  tunnel: w358 -> [w375]
                  tunnel: [w370] -> w342
                  tunnel: [w369] -> w344
                  shift-right: [w371] -> w348
                  shift-left: w353 -> [w372]
                  n117 = call "ADIS16448 Scale Data.vi"("error in (no error)"=w375, "New Data In"=w376) -> ("error out"=w369:errorcluster, "Data Good?"=w374:bool, "Data Out"=w373:dbl[])  [unwired: 7 in]
                  n118 = case shown="True" w374 {
                    tunnel: w373 -> [w378 w380]
                    tunnel: [w378 w379] -> w370
                    tunnel: w372 -> [w377 w388]
                    tunnel: [w377 w387] -> w371
                    frame False {
                    }
                    frame True {
                      n119 = Index Array(array=w380) -> (element #1=w381:dbl, element #2=w382:dbl, element #3=w383:dbl)  [unwired: 3 in]
                      n120 = Increment(x=w388) -> (x+1=w387:i32)
                      n121 = call <vilib>:"Mean PtByPt.vi"("x"=w381) -> ("mean"=w384:dbl)  [unwired: 3 in, 1 out]
                      n122 = call <vilib>:"Mean PtByPt.vi"("x"=w382) -> ("mean"=w385:dbl)  [unwired: 3 in, 1 out]
                      n123 = call <vilib>:"Mean PtByPt.vi"("x"=w383) -> ("mean"=w386:dbl)  [unwired: 3 in, 1 out]
                      n124 = Build Array(w384, w385, w386) -> (w379:dbl[])
                    }
                  }
                }
                n125 = Greater?(x=w348, y=w352) -> (0:w351:bool)
                n126 = case shown="True" w351 {
                  tunnel: w348 -> [w363 _]
                  tunnel: [w363 0 ("Offset Counter")] -> w347
                  tunnel: w346 -> [w362 w367]
                  tunnel: w344 -> [w361 w365]
                  tunnel: [w361 w365] -> w343
                  frame False {
                    n127 = RT FIFO Write(0:w362, 1:T17 {"Command"=enum."Recalibrate", "Data"=0} ("element")) -> ()  [unwired: 3 in, 4 out]
                  }
                  frame True {
                    n128 = RT FIFO Write(0:w367, 1:T17 {"Command"=enum."Recal Complete", "Data"=0} ("element")) -> ()  [unwired: 3 in, 4 out]
                  }
                }
                n129 = Bundle By Name(cluster=w350, "Offset Counter"=w347, "Offsets"=w342) -> (w349:T14)
              }
            }
          }
          frame "Recal Complete" {
            n130 = Send Notification(notification="", notifier=w397) -> ()  [unwired: 1 in, 2 out]
            n131 = RT FIFO Write(0:w395, 1:T15 {"Calibrated?"=TRUE} ("element")) -> ()  [unwired: 3 in, 4 out]
            n132 = Bundle By Name(cluster=w393, "AutoSPI Override"=FALSE, "AutoSPI Active?"=TRUE, "Reset"=TRUE) -> (w392:T14)
          }
          frame "Exit Auto SPI" {
            w417 = T16 114 items=["Reserved1"=0, "DIAG_STAT"=2, "X_GYRO_LOW"=4, "X_GYRO_OUT"=6, "Y_GYRO_LOW"=8, "Y_GYRO_OUT"=10, "Z_GYRO_LOW"=12, "Z_GYRO_OUT"=14, "X_ACCL_LOW"=16, "X_ACCL_OUT"=18, "Y_ACCL_LOW"=20, "Y_ACCL_OUT"=22, "Z_ACCL_LOW"=24, "Z_ACCL_OUT"=26, "TEMP_OUT"=28, "TIME_STAMP"=30, "Reseved2"=32, "DATA_CNTR"=34, "X_DELTANG_LOW"=36, "X_DELTANG_OUT"=38, "Y_DELTANG_LOW"=40, "Y_DELTANG_OUT"=42, "Z_DELTANG_LOW"=44, "Z_DELTANG_OUT"=46, "X_DELTVEL_LOW"=48, "X_DELTVEL_OUT"=50, "Y_DELTVEL_LOW"=52, "Y_DELTVEL_OUT"=54, "Z_DELTVEL_LOW"=56, "Z_DELTVEL_OUT"=58, "Reserved3"=60, "Reserved4"=62, "XG_BIAS_LOW"=64, "XG_BIAS_HIGH"=66, "YG_BIAS_LOW"=68, "YG_BIAS_OUT"=70, "ZG_BIAS_LOW"=72, "ZG_BIAS_OUT"=74, "XA_BIAS_LOW"=76, "XA_BIAS_HIGH"=78, "YA_BIAS_LOW"=80, "YA_BIAS_OUT"=82, "ZA_BIAS_LOW"=84, "ZA_BIAS_OUT"=86, "Reserved5"=88, "Reserved6"=90, "FILT_CTRL"=92, "Reserved5"=94, "MSC_CTRL"=96, "UP_SCALE"=98, "DEC_RATE"=100, "NULL_CNFG"=102, "GLOB_CMD"=104, "Reserved6"=106, "FIRM_REV"=108, "FIRM_DM"=110, "FIRM_Y"=112, "PROD_ID"=114, "SERIAL_NUM"=116, "USER_SCR1"=118, "USER_SCR2"=120, "USER_SCR3"=122, "FLSHCNT_LOW"=124, "FLSHCNT_HIGH"=126] ("ADIS16448 Register")
            n133 = Unbundle By Name(w404) -> ("ADIS16448DevRef.Hardware Config.IMU SPI Bus"=w420:T7, "ADIS16448DevRef.Hardware Config.SPI Clock Rate (Hz)"=w419:dbl, "ADIS16448DevRef.Hardware Config.IMU SPI Mode (3)"=w418:T5, "SPIDevRef"=w399:T13)
            n134 = call <vilib>:"WPI_SPIClose.vi"("error in (no error)"=w423, "SPIDevRef"=w399) -> ("error out"=w408:errorcluster)  [unwired: 9 in]
            n135 = call <vilib>:"WPI_DigitalOutputRefNum Registry Get.vi"("error in (no error)"=w408, "refnum name"="448 Status LED") -> ("error out"=w402:errorcluster, "DigitalOutputDevRef"=w401:T18)  [unwired: 8 in]
            n136 = RT FIFO Write(0:w421, 1:T17 {"Command"=enum."Rewrite Config", "Data"=0} ("element")) -> ()  [unwired: 3 in, 4 out]
            n137 = call <vilib>:"WPI_DigitalOutputSetValue.vi"("error in (no error)"=w402, "Value"=TRUE, "DigitalOutputDevRef"=w401) -> ("error out"=w403:errorcluster)  [unwired: 7 in, 1 out]
            n138 = call <vilib>:"WPI_SPIOpen.vi"("error in"=w403, "Mode (3)"=w418, "Clock Rate (Hz)"=w419, "SPI Bus"=w420) -> ("error out"=w416:errorcluster, "SPIDevRef"=w412:T13)  [unwired: 6 in]
            n139 = call "ADIS16448 Read Register.vi"("error in (no error)"=w416, "ADIS16448 Register"=w417, "SPIDevRef in"=w412) -> ("error out"=w413:errorcluster, "Register Value"=w411:u16, "SPIDevRef out"=w414:T13)  [unwired: 6 in]
            n140 = Equal?(x=u16 16448 ("y"), y=w411) -> (x = y?=w415:bool)
            n141 = case shown="True" w415 {
              tunnel: w414 -> [_ w437]
              tunnel: w413 -> [w426 w436]
              tunnel: [w425 w435] -> w410
              tunnel: w407 -> [w424 w433]
              tunnel: [w424 w432] -> w406
              frame False {
                n142 = case shown="No Error" w426 {
                  selector: w426 -> [w428 w431]
                  tunnel: [w427 w431] -> w425
                  frame No Error {
                    n143 = call <vilib>:"Error Cluster From Error Code.vi"("error in (no error)"=w428, "error message (\"\")"="SPI port did not reset properly" ("error message (\"\")"), "error code (0)"=-8106) -> ("error out"=w427:errorcluster)  [unwired: 6 in]
                  }
                  frame Error {
                  }
                }
              }
              frame True {
                n144 = call <vilib>:"WPI_SPIRefNum Registry Set.vi"("error in (no error)"=w436, "refnum name"="AutoSPI", "SPIDevRef"=w437) -> ("error out"=w435:errorcluster, "SPIDevRef"=w438:T13)  [unwired: 7 in]
                n145 = Bundle By Name(cluster=w433, "SPIDevRef"=w438, "AutoSPI Active?"=FALSE) -> (w432:T14)
              }
            }
          }
          frame "Start Auto SPI" {
            n146 = Unbundle By Name(w445) -> ("SPIDevRef"=w444:T13, "Digital Source"=w443:T9, "ADIS16448DevRef.Hardware Config.Stall Config"=w442:T20, "Data Header"=w441:u8[], "Zero Byte Count"=w440:u8)
            n147 = Unbundle By Name(w444) -> ("SPI Bus"=w457:T7)
            n148 = RT FIFO Write(0:w458, 1:T17 {"Command"=enum."Recal Complete", "Data"=0} ("element")) -> ()  [unwired: 3 in, 4 out]
            n149 = call <vilib>:"FPGA_SPI_ConfigureAuto.vi"("SPI Auto Zero Byte Count"=w440, "error in"=w456, "SPI Auto TX Byte Array"=w441, "Stall Config"=w442, "SPI Bus"=w457) -> ("error out"=w449:errorcluster)  [unwired: 6 in]
            n150 = call <vilib>:"FPGA_SPI_StartAuto_External.vi"("error in (no error)"=w449, "Falling Edge"=FALSE, "Rising Edge"=TRUE, "Source"=w443) -> ("error out"=w453:errorcluster)  [unwired: 7 in]
            n151 = call <vilib>:"WPI_DigitalOutputRefNum Registry Get.vi"("error in (no error)"=w453, "refnum name"="448 Status LED") -> ("error out"=w452:errorcluster, "DigitalOutputDevRef"=w451:T18)  [unwired: 8 in]
            n152 = call <vilib>:"WPI_DigitalOutputSetValue.vi"("error in (no error)"=w452, "Value"=FALSE, "DigitalOutputDevRef"=w451) -> ("error out"=w447:errorcluster)  [unwired: 7 in, 1 out]
          }
          frame "Start Recal" {
            n153 = RT FIFO Write(0:w463, 1:T15 {"Calibrated?"=FALSE} ("element")) -> ()  [unwired: 3 in, 4 out]
            n154 = Bundle By Name(cluster=w461, "AutoSPI Override"=TRUE) -> (w460:T14)
          }
        }
      }
    }
  }
  n155 = while {
    tunnel: w8 -> [w467]
    tunnel: [w466] -> w2
    stop <- w466 stop-if-true
    # "stop this VI when the VI calling StartComm goes idle"
    n156 = property class="VI"(reference=w467) -> ("Exec.State"=w469:T22)  [unwired: 1 in, 2 out]
    n157 = Wait (ms)(milliseconds to wait=u32 250) -> ()  [unwired: 1 out]
    n158 = Equal?(x=w469, y=T22."Idle" ("Execution:State")) -> (x = y?=w466:bool)
  }
  n159 = flat-sequence {
    tunnel: w2 -> [_]
    frame #0 {
      n160 = call <vilib>:"WPI_DigitalOutputRefNum Registry Get.vi"("refnum name"="448 Status LED") -> ("error out"=w476:errorcluster, "DigitalOutputDevRef"=w475:T18)  [unwired: 9 in]
      n161 = call <vilib>:"WPI_DigitalOutputClose.vi"("error in (no error)"=w476, "DigitalOutputDevRef"=w475) -> ("error out"=w471:errorcluster)  [unwired: 9 in]
      n162 = call <vilib>:"WPI_SPIRefNum Registry Get.vi"("error in (no error)"=w471, "refnum name"="AutoSPI") -> ("error out"=w473:errorcluster, "SPIDevRef"=w472:T13)  [unwired: 8 in]
      n163 = call <vilib>:"WPI_SPIClose.vi"("error in (no error)"=w473, "SPIDevRef"=w472) -> ()  [unwired: 9 in, 1 out]
    }
    frame #1 {
      n164 = Stop() -> ()  [unwired: 1 in]
    }
  }
